vi "Prueba Tension.vi"(11 "Class 2.lvclass":refnum<class "Class 2.lvclass">) -> (3 "Class 2.lvclass 2":refnum<class "Class 2.lvclass">)   [LabVIEW 2019, in "Class 2.lvclass"]
uses:
  Class 2.lvclass
  Class 2.lvclass/Class 2.ctl
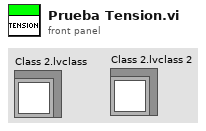
[diagram p1: front panel]
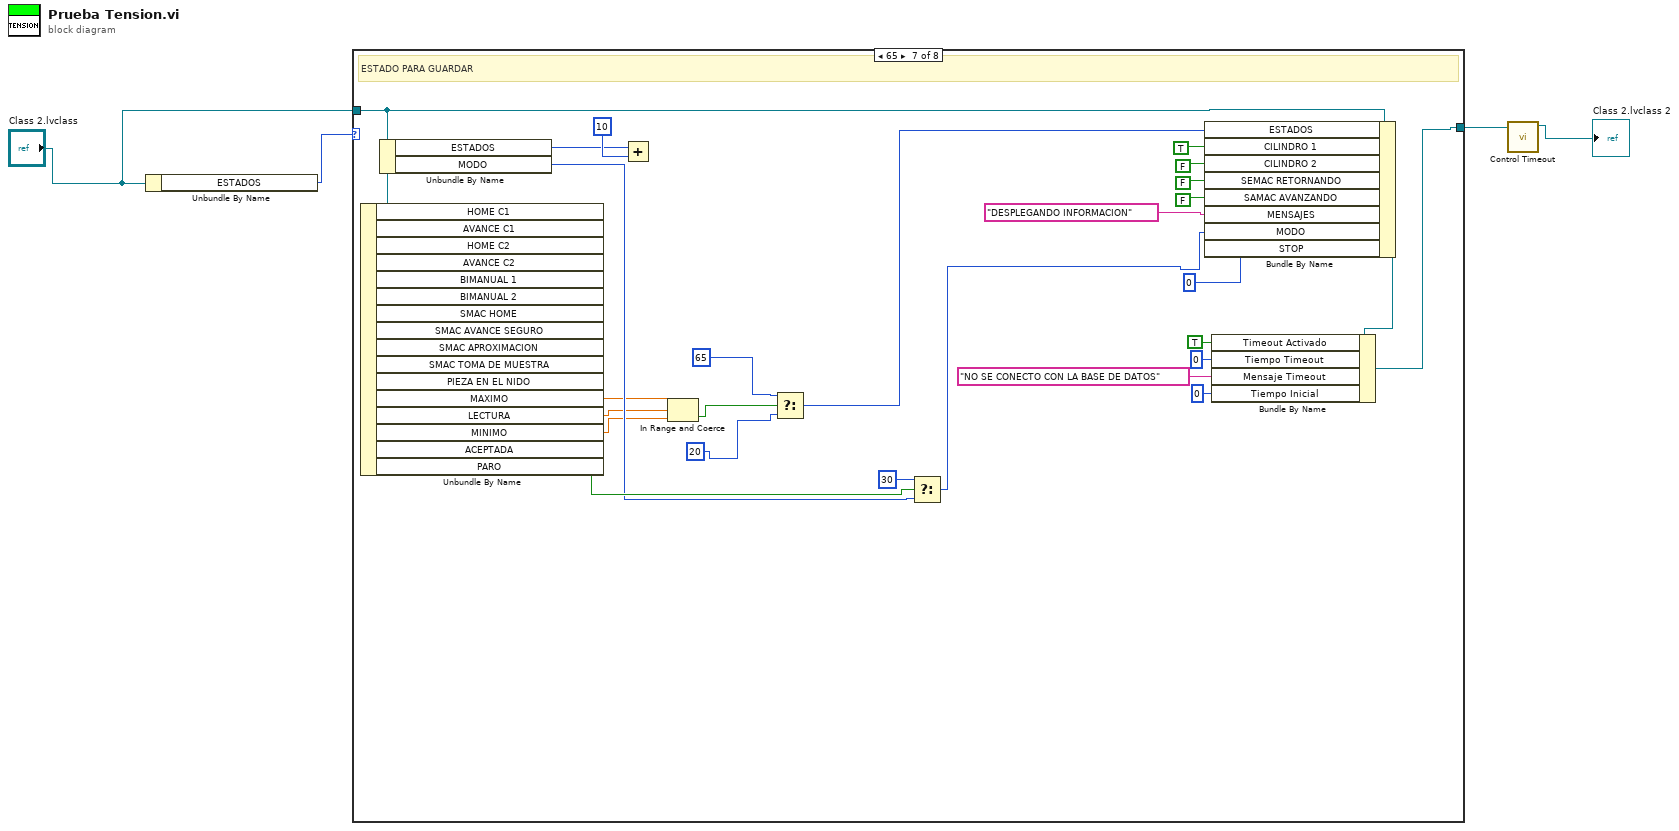
[diagram p0: block diagram]
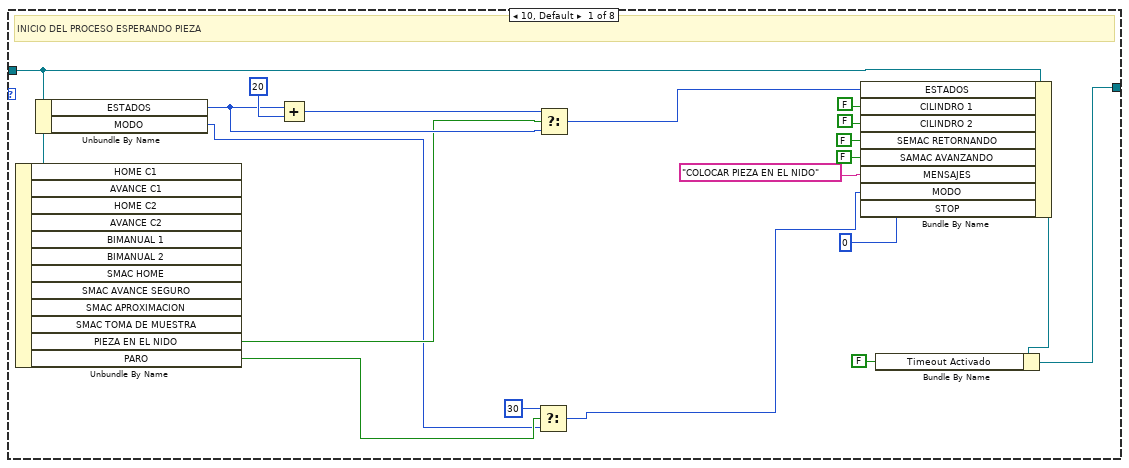
[diagram p2: hidden frame]
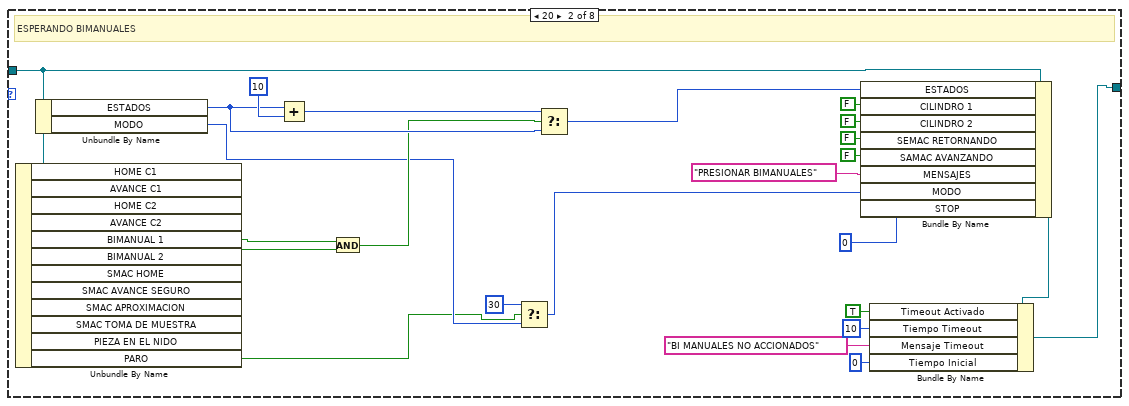
[diagram p3: hidden frame]
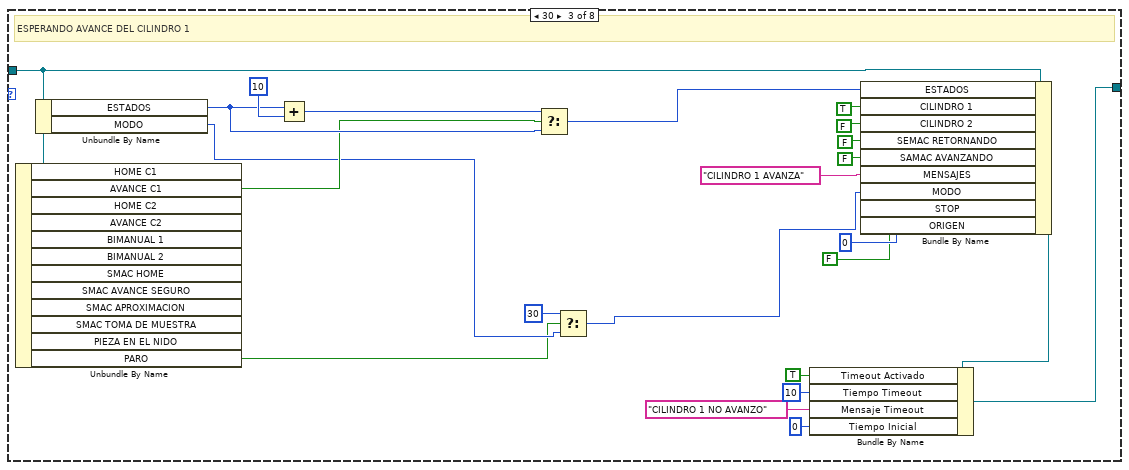
[diagram p4: hidden frame]
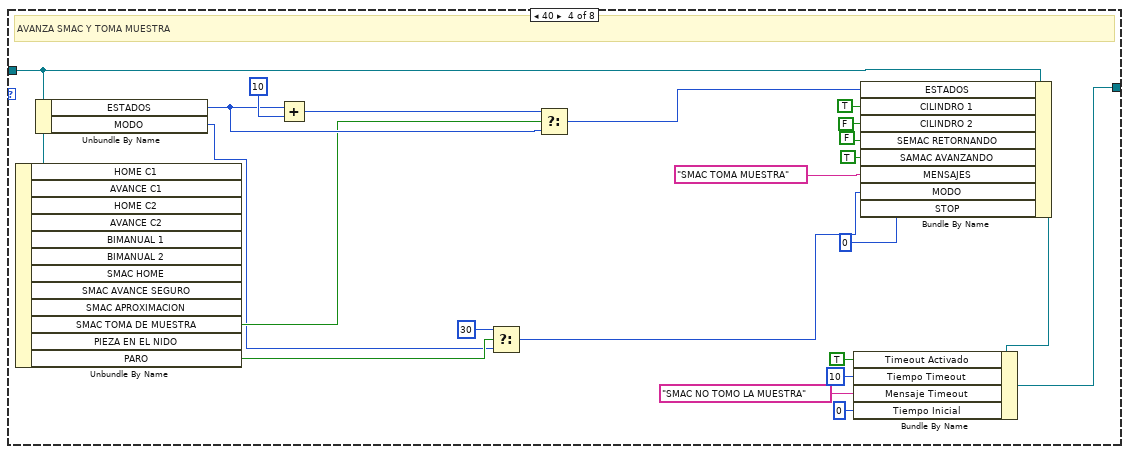
[diagram p5: hidden frame]
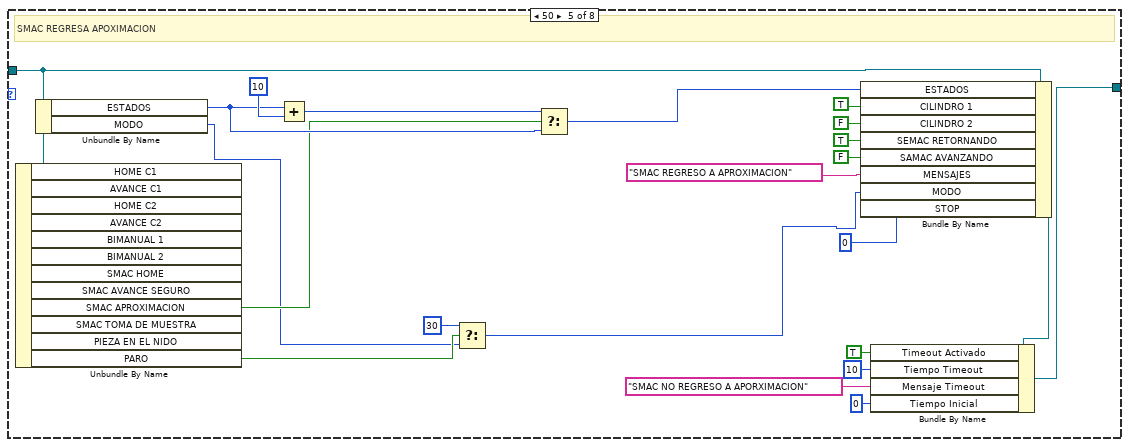
[diagram p6: hidden frame]
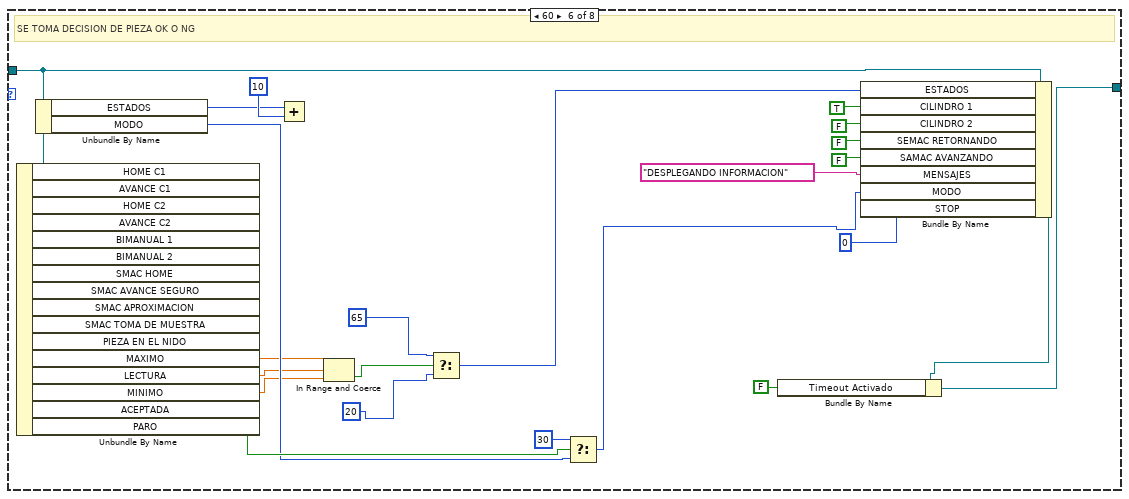
[diagram p7: hidden frame]
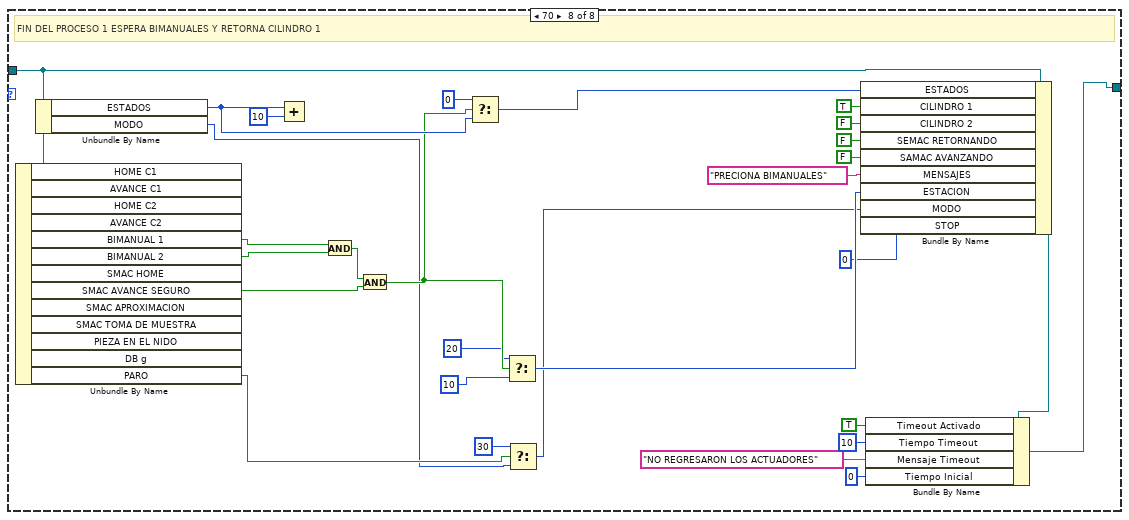
[diagram p8: hidden frame]
diagram:
  n1 = Unbundle By Name("Class 2.lvclass") -> ("ESTADOS"=w4:i16)
  n2 = case shown="65" w4 {
    tunnel: "Class 2.lvclass" -> [w19 w43 w66 w88 w110 w136 w162 w191]
    tunnel: [w5 w24 w48 w71 w94 w115 w138 w164] -> w2
    frame 10, Default {
      # "INICIO DEL PROCESO ESPERANDO PIEZA"
      n3 = Unbundle By Name(w19) -> ("PIEZA EN EL NIDO"=w17:bool, "PARO"=w11:bool)  [unwired: 10 out]
      n4 = Unbundle By Name(w19) -> ("ESTADOS"=w21:i16, "MODO"=w10:i16)
      n5 = Add(x=w21, y=i16 20) -> (x+y=w22:i16)
      n6 = Select(t=i16 30, s=w11, f=w10) -> (s? t:f=w9:i16)
      n7 = Select(t=w22, s=w17, f=w21) -> (s? t:f=w20:i16)
      n8 = Bundle By Name(cluster=w19, "ESTADOS"=w20, "CILINDRO 1"=FALSE ("SALIDAS.CILINDRO 1"), "CILINDRO 2"=FALSE ("SALIDAS.CILINDRO 2"), "SEMAC RETORNANDO"=FALSE ("SALIDAS.SEMAC RETORNANDO"), "SAMAC AVANZANDO"=FALSE ("SALIDAS.SAMAC AVANZANDO"), "MENSAJES"="COLOCAR PIEZA EN EL NIDO" ("SALIDAS.MENSAJES"), "MODO"=w9, "STOP"=i16 0 ("MAQ DE ESTADOS.STOP")) -> (w6:refnum<class "Class 2.lvclass">)
      n9 = Bundle By Name(cluster=w6, "Timeout Activado"=FALSE ("Timeout.Timeout Activado")) -> (w5:refnum<class "Class 2.lvclass">)
    }
    frame 20 {
      # "ESPERANDO BIMANUALES"
      n10 = Unbundle By Name(w43) -> ("BIMANUAL 1"=w37:bool, "BIMANUAL 2"=w36:bool, "PARO"=w32:bool)  [unwired: 9 out]
      n11 = Unbundle By Name(w43) -> ("ESTADOS"=w45:i16, "MODO"=w33:i16)
      n12 = Add(x=w45, y=i16 10) -> (x+y=w46:i16)
      n13 = And(x=w37, y=w36) -> (x .and. y?=w35:bool)
      n14 = Select(t=i16 30, s=w32, f=w33) -> (s? t:f=w31:i16)
      n15 = Select(t=w46, s=w35, f=w45) -> (s? t:f=w44:i16)
      n16 = Bundle By Name(cluster=w43, "ESTADOS"=w44, "CILINDRO 1"=FALSE ("SALIDAS.CILINDRO 1"), "CILINDRO 2"=FALSE ("SALIDAS.CILINDRO 2"), "SEMAC RETORNANDO"=FALSE ("SALIDAS.SEMAC RETORNANDO"), "SAMAC AVANZANDO"=FALSE ("SALIDAS.SAMAC AVANZANDO"), "MENSAJES"="PRESIONAR BIMANUALES" ("SALIDAS.MENSAJES"), "MODO"=w31, "STOP"=i16 0 ("MAQ DE ESTADOS.STOP")) -> (w25:refnum<class "Class 2.lvclass">)
      n17 = Bundle By Name(cluster=w25, "Timeout Activado"=TRUE ("Timeout.Timeout Activado"), "Tiempo Timeout"=u32 10 ("Timeout.Tiempo Timeout"), "Mensaje Timeout"="BI MANUALES NO ACCIONADOS" ("Timeout.Mensaje Timeout"), "Tiempo Inicial"=u32 0 ("Timeout.Tiempo Inicial")) -> (w24:refnum<class "Class 2.lvclass">)
    }
    frame 30 {
      # "ESPERANDO AVANCE DEL CILINDRO 1"
      n18 = Unbundle By Name(w66) -> ("AVANCE C1"=w60:bool, "PARO"=w55:bool)  [unwired: 10 out]
      n19 = Unbundle By Name(w66) -> ("ESTADOS"=w68:i16, "MODO"=w56:i16)
      n20 = Add(x=w68, y=i16 10) -> (x+y=w69:i16)
      n21 = Select(t=w69, s=w60, f=w68) -> (s? t:f=w67:i16)
      n22 = Select(t=i16 30, s=w55, f=w56) -> (s? t:f=w58:i16)
      n23 = Bundle By Name(cluster=w66, "ESTADOS"=w67, "CILINDRO 1"=TRUE ("SALIDAS.CILINDRO 1"), "CILINDRO 2"=FALSE ("SALIDAS.CILINDRO 2"), "SEMAC RETORNANDO"=FALSE ("SALIDAS.SEMAC RETORNANDO"), "SAMAC AVANZANDO"=FALSE ("SALIDAS.SAMAC AVANZANDO"), "MENSAJES"="CILINDRO 1 AVANZA" ("SALIDAS.MENSAJES"), "MODO"=w58, "STOP"=i16 0 ("MAQ DE ESTADOS.STOP"), "ORIGEN"=FALSE ("PROCESO.ORIGEN")) -> (w49:refnum<class "Class 2.lvclass">)
      n24 = Bundle By Name(cluster=w49, "Timeout Activado"=TRUE ("Timeout.Timeout Activado"), "Tiempo Timeout"=u32 10 ("Timeout.Tiempo Timeout"), "Mensaje Timeout"="CILINDRO 1 NO AVANZO" ("Timeout.Mensaje Timeout"), "Tiempo Inicial"=u32 0 ("Timeout.Tiempo Inicial")) -> (w48:refnum<class "Class 2.lvclass">)
    }
    frame 40 {
      # "AVANZA SMAC Y TOMA MUESTRA"
      n25 = Unbundle By Name(w88) -> ("SMAC TOMA DE MUESTRA"=w82:bool, "PARO"=w80:bool)  [unwired: 10 out]
      n26 = Unbundle By Name(w88) -> ("ESTADOS"=w90:i16, "MODO"=w79:i16)
      n27 = Add(x=w90, y=i16 10) -> (x+y=w91:i16)
      n28 = Select(t=i16 30, s=w80, f=w79) -> (s? t:f=w78:i16)
      n29 = Select(t=w91, s=w82, f=w90) -> (s? t:f=w89:i16)
      n30 = Bundle By Name(cluster=w88, "ESTADOS"=w89, "CILINDRO 1"=TRUE ("SALIDAS.CILINDRO 1"), "CILINDRO 2"=FALSE ("SALIDAS.CILINDRO 2"), "SEMAC RETORNANDO"=FALSE ("SALIDAS.SEMAC RETORNANDO"), "SAMAC AVANZANDO"=TRUE ("SALIDAS.SAMAC AVANZANDO"), "MENSAJES"="SMAC TOMA MUESTRA" ("SALIDAS.MENSAJES"), "MODO"=w78, "STOP"=i16 0 ("MAQ DE ESTADOS.STOP")) -> (w72:refnum<class "Class 2.lvclass">)
      n31 = Bundle By Name(cluster=w72, "Timeout Activado"=TRUE ("Timeout.Timeout Activado"), "Tiempo Timeout"=u32 10 ("Timeout.Tiempo Timeout"), "Mensaje Timeout"="SMAC NO TOMO LA MUESTRA" ("Timeout.Mensaje Timeout"), "Tiempo Inicial"=u32 0 ("Timeout.Tiempo Inicial")) -> (w71:refnum<class "Class 2.lvclass">)
    }
    frame 50 {
      # "SMAC REGRESA APOXIMACION"
      n32 = Unbundle By Name(w110) -> ("SMAC APROXIMACION"=w104:bool, "PARO"=w102:bool)  [unwired: 10 out]
      n33 = Unbundle By Name(w110) -> ("ESTADOS"=w112:i16, "MODO"=w101:i16)
      n34 = Add(x=w112, y=i16 10) -> (x+y=w113:i16)
      n35 = Select(t=i16 30, s=w102, f=w101) -> (s? t:f=w100:i16)
      n36 = Select(t=w113, s=w104, f=w112) -> (s? t:f=w111:i16)
      n37 = Bundle By Name(cluster=w110, "ESTADOS"=w111, "CILINDRO 1"=TRUE ("SALIDAS.CILINDRO 1"), "CILINDRO 2"=FALSE ("SALIDAS.CILINDRO 2"), "SEMAC RETORNANDO"=TRUE ("SALIDAS.SEMAC RETORNANDO"), "SAMAC AVANZANDO"=FALSE ("SALIDAS.SAMAC AVANZANDO"), "MENSAJES"="SMAC REGRESO A APROXIMACION" ("SALIDAS.MENSAJES"), "MODO"=w100, "STOP"=i16 0 ("MAQ DE ESTADOS.STOP")) -> (w95:refnum<class "Class 2.lvclass">)
      n38 = Bundle By Name(cluster=w95, "Timeout Activado"=TRUE ("Timeout.Timeout Activado"), "Tiempo Timeout"=u32 10 ("Timeout.Tiempo Timeout"), "Mensaje Timeout"="SMAC NO REGRESO A APORXIMACION" ("Timeout.Mensaje Timeout"), "Tiempo Inicial"=u32 0 ("Timeout.Tiempo Inicial")) -> (w94:refnum<class "Class 2.lvclass">)
    }
    frame 60 {
      # "SE TOMA DECISION DE PIEZA OK O NG"
      n39 = Unbundle By Name(w136) -> ("MAXIMO"=w121:dbl, "LECTURA"=w119:dbl, "MINIMO"=w120:dbl, "PARO"=w126:bool)  [unwired: 12 out]
      n40 = Unbundle By Name(w136) -> ("ESTADOS"=w130:i16, "MODO"=w125:i16)
      n41 = Add(x=w130, y=i16 10) -> ()  [unwired: 1 out]
      n42 = In Range and Coerce(upper limit=w121, x=w119, lower limit=w120) -> (In Range?=w124:bool)  [unwired: 1 out]
      n43 = Select(t=i16 65 ("y"), s=w124, f=i16 20 ("y")) -> (s? t:f=w118:i16)
      n44 = Select(t=i16 30, s=w126, f=w125) -> (s? t:f=w128:i16)
      n45 = Bundle By Name(cluster=w136, "ESTADOS"=w118, "CILINDRO 1"=TRUE ("SALIDAS.CILINDRO 1"), "CILINDRO 2"=FALSE ("SALIDAS.CILINDRO 2"), "SEMAC RETORNANDO"=FALSE ("SALIDAS.SEMAC RETORNANDO"), "SAMAC AVANZANDO"=FALSE ("SALIDAS.SAMAC AVANZANDO"), "MENSAJES"="DESPLEGANDO INFORMACION" ("SALIDAS.MENSAJES"), "MODO"=w128, "STOP"=i16 0 ("MAQ DE ESTADOS.STOP")) -> (w116:refnum<class "Class 2.lvclass">)
      n46 = Bundle By Name(cluster=w116, "Timeout Activado"=FALSE ("Timeout.Timeout Activado")) -> (w115:refnum<class "Class 2.lvclass">)
    }
    frame 65 {
      # "ESTADO PARA GUARDAR"
      n47 = Unbundle By Name(w162) -> ("MAXIMO"=w147:dbl, "LECTURA"=w145:dbl, "MINIMO"=w146:dbl, "PARO"=w152:bool)  [unwired: 12 out]
      n48 = Unbundle By Name(w162) -> ("ESTADOS"=w156:i16, "MODO"=w151:i16)
      n49 = Add(x=w156, y=i16 10) -> ()  [unwired: 1 out]
      n50 = In Range and Coerce(upper limit=w147, x=w145, lower limit=w146) -> (In Range?=w150:bool)  [unwired: 1 out]
      n51 = Select(t=i16 65 ("y"), s=w150, f=i16 20 ("y")) -> (s? t:f=w144:i16)
      n52 = Select(t=i16 30, s=w152, f=w151) -> (s? t:f=w154:i16)
      n53 = Bundle By Name(cluster=w162, "ESTADOS"=w144, "CILINDRO 1"=TRUE ("SALIDAS.CILINDRO 1"), "CILINDRO 2"=FALSE ("SALIDAS.CILINDRO 2"), "SEMAC RETORNANDO"=FALSE ("SALIDAS.SEMAC RETORNANDO"), "SAMAC AVANZANDO"=FALSE ("SALIDAS.SAMAC AVANZANDO"), "MENSAJES"="DESPLEGANDO INFORMACION" ("SALIDAS.MENSAJES"), "MODO"=w154, "STOP"=i16 0 ("MAQ DE ESTADOS.STOP")) -> (w139:refnum<class "Class 2.lvclass">)
      n54 = Bundle By Name(cluster=w139, "Timeout Activado"=TRUE ("Timeout.Timeout Activado"), "Tiempo Timeout"=u32 0 ("Timeout.Tiempo Timeout"), "Mensaje Timeout"="NO SE CONECTO CON LA BASE DE DATOS" ("Timeout.Mensaje Timeout"), "Tiempo Inicial"=u32 0 ("Timeout.Tiempo Inicial")) -> (w138:refnum<class "Class 2.lvclass">)
    }
    frame 70 {
      # "FIN DEL PROCESO 1 ESPERA BIMANUALES Y RETORNA CILINDRO 1"
      n55 = Unbundle By Name(w191) -> ("BIMANUAL 1"=w183:bool, "BIMANUAL 2"=w182:bool, "SMAC AVANCE SEGURO"=w179:bool, "PARO"=w171:bool)  [unwired: 9 out]
      n56 = Unbundle By Name(w191) -> ("ESTADOS"=w184:i16, "MODO"=w170:i16)
      n57 = Add(x=w184, y=i16 10) -> ()  [unwired: 1 out]
      n58 = And(x=w183, y=w182) -> (x .and. y?=w180:bool)
      n59 = And(x=w180, y=w179) -> (x .and. y?=w178:bool)
      n60 = Select(t=i16 0, s=w178, f=w184) -> (s? t:f=w185:i16)
      n61 = Select(t=i16 20, s=w178, f=i16 10 ("t")) -> (s? t:f=w175:i16)
      n62 = Select(t=i16 30, s=w171, f=w170) -> (s? t:f=w173:i16)
      n63 = Bundle By Name(cluster=w191, "ESTADOS"=w185, "CILINDRO 1"=TRUE ("SALIDAS.CILINDRO 1"), "CILINDRO 2"=FALSE ("SALIDAS.CILINDRO 2"), "SEMAC RETORNANDO"=FALSE ("SALIDAS.SEMAC RETORNANDO"), "SAMAC AVANZANDO"=FALSE ("SALIDAS.SAMAC AVANZANDO"), "MENSAJES"="PRECIONA BIMANUALES" ("SALIDAS.MENSAJES"), "ESTACION"=w175, "MODO"=w173, "STOP"=i16 0 ("MAQ DE ESTADOS.STOP")) -> (w165:refnum<class "Class 2.lvclass">)
      n64 = Bundle By Name(cluster=w165, "Timeout Activado"=TRUE ("Timeout.Timeout Activado"), "Tiempo Timeout"=u32 10 ("Timeout.Tiempo Timeout"), "Mensaje Timeout"="NO REGRESARON LOS ACTUADORES" ("Timeout.Mensaje Timeout"), "Tiempo Inicial"=u32 0 ("Timeout.Tiempo Inicial")) -> (w164:refnum<class "Class 2.lvclass">)
    }
  }
  n65 = call "Control Timeout.vi"("Class 2 in"=w2) -> ("Class 2 out"=→"Class 2.lvclass 2":refnum<class "Class 2.lvclass">)  [unwired: 10 in]
